vi "_Static Data (Global).vi"() -> ()   [LabVIEW 2009, in "Numeric Test Object.lvclass"]
doc: "This global variable is used to implement static data."
uses:
  Numeric Test Object.lvclass
panel:
  in  "Static Int":i32
  # "By using a global vi as a private member of the class, this becomes a static variable that is shared among all class instances."
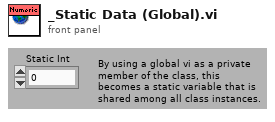
[diagram p1: front panel]
diagram:
